vi "Write DefBallTrajSkill.vi"(8 "error in (no error)":errorcluster, 10 "DefBallTrajSkill":refnum<class "DefBallTrajSkill.lvclass">, 11 "Skillbook in":refnum<class "Skillbook.lvclass">) -> (0 "error out":errorcluster, 3 "Skillbook out":refnum<class "Skillbook.lvclass">)   [LabVIEW 2023, in "Skillbook.lvclass"]
uses:
  Skillbook.lvclass
  DefBallTrajSkill_class/DefBallTrajSkill.lvclass
  Skillbook.lvclass/Skillbook.ctl
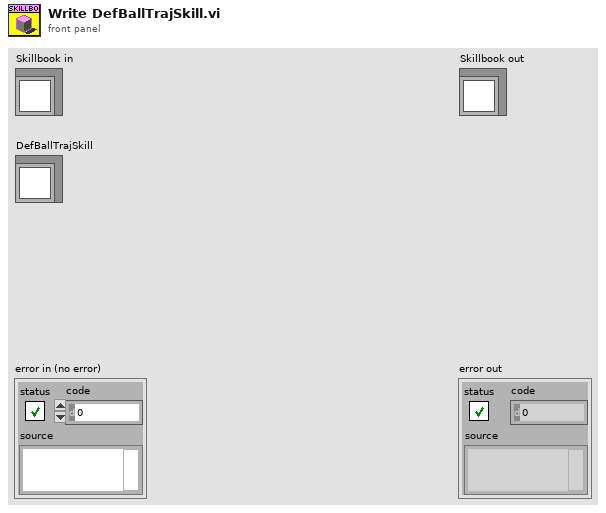
[diagram p1: front panel]
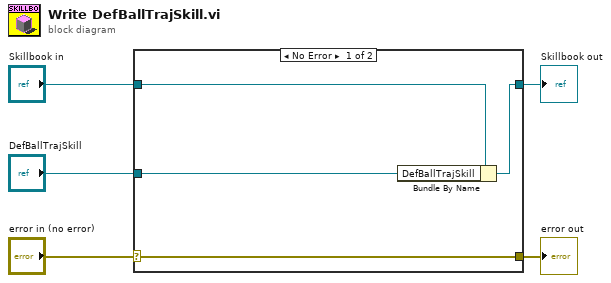
[diagram p0: block diagram]
diagram:
  n1 = case shown="No Error" "error in (no error)" {
    selector: "error in (no error)" -> [w9 w10]
    tunnel: [w9 w10] -> w4
    tunnel: [w7 w11] -> w2
    tunnel: "Skillbook in" -> [w8 w11]
    tunnel: "DefBallTrajSkill" -> [w6 _]
    frame No Error {
      n2 = Bundle By Name(cluster=w8, "DefBallTrajSkill"=w6) -> (w7:refnum<class "Skillbook.lvclass">)
    }
    frame Error {
    }
  }
  "error out" <- w4
  "Skillbook out" <- w2
